vi "Upload.vi"(8 "error in":errorcluster, 9 "Multiplexer":cluster{"Index":u16, "Sub-Index":u8} {"Index" format="%04x"; "Sub-Index" format="%.0x"}, 10 "Node-ID":u8, 11 "CANopen Master in":refnum<class "CANopen Master.lvclass">) -> (0 "error out":errorcluster, 1 "Value":u8[](array[numeric]), 2 "Success?":bool, 3 "CANopen Master out":refnum<class "CANopen Master.lvclass">)   [LabVIEW 2024, in "CANopen Master.lvclass"]
uses:
  CANopen Master.lvclass
  CANopen Master.lvclass/CANopen Master.ctl
  HAL/Source/Interfaces/ICommunicate/ICommunicate.lvclass
  SDO Manager/SDO Manager.lvclass
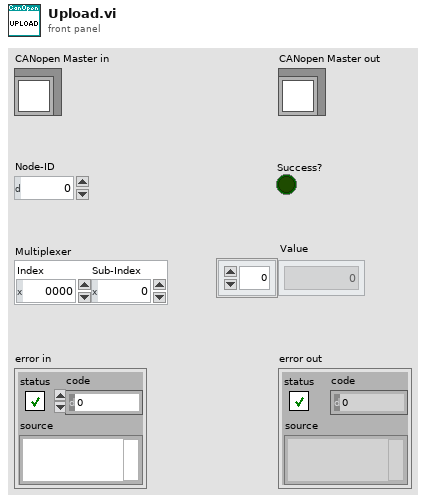
[diagram p1: front panel]
types:
  T1 = typedef "CANopen.lvlib/SDO Result.ctl" = cluster{"Success":bool, "SDO abort code":cluster{"Null":bool, "Value":T2}, "Data":cluster{"Null":bool, "Data":u8[]}}
  T2 = typedef "CANopen Master.lvlib/SDO Transfer.lvclass/SDO abort code.ctl" = u32
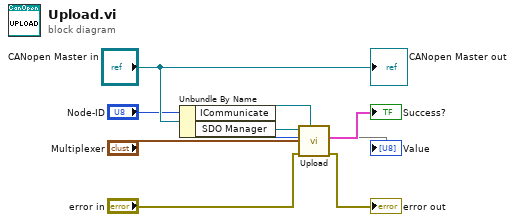
[diagram p0: block diagram]
diagram:
  n1 = Unbundle By Name("CANopen Master in") -> ("ICommunicate"=w5:refnum<class "ICommunicate.lvclass">, "SDO Manager"=w6:refnum<class "SDO Manager.lvclass">)
  n2 = call "Upload.vi"(7:w5, "Error In"="error in", "Timeout"="Multiplexer", "Parameters"="Node-ID", "SDO Manager in"=w6) -> ("Error Out"=→"error out":errorcluster, 1:→"Value", "SDO Result"=→"Success?":T1)  [unwired: 3 in, 1 out]
  "CANopen Master out" <- "CANopen Master in"
